vi "TCP Engine Send Loop.vi"(8 "error in (no error)":errorcluster, 11 "Send Loop Notifier":refnum<notifier>) -> (0 "error out":errorcluster)   [LabVIEW 2024, in "TCP Engine.lvlib"]
doc: "This VI will semd all engine response to HOST\n\n\n\nAll Rights Reserved © 2017 SyncSols"
uses:
  TCP Engine.lvlib
  Controls/TCP Engine Send Loop State Machine Data Cluster.ctl
  Controls/TCP Engine Send Loop Data.ctl
  Controls/TCP Engine Send Loop State Machine Cases.ctl
  Main Engine/Controls/Main Engine Q Option.ctl
  Controls/TCP Engine Q Driver Options.ctl
  Controls/TCP Engine State Machine Cases.ctl
panel:
  in  "Data Cluster":T1
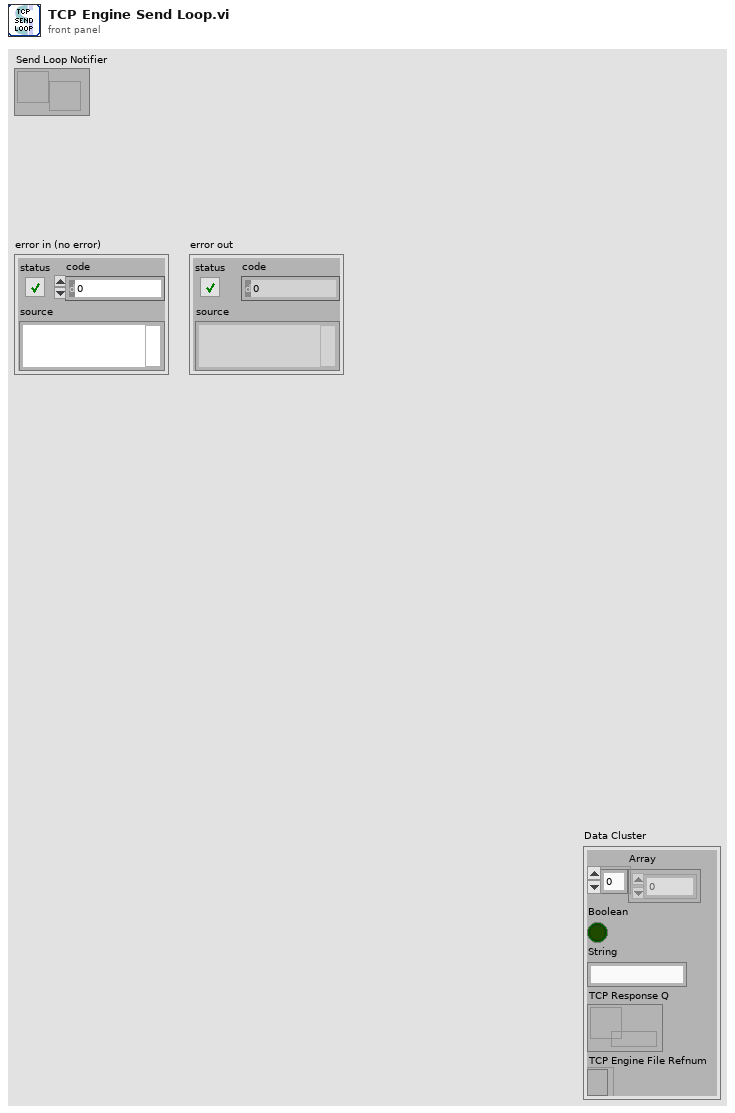
[diagram p1: front panel]
types:
  T1 = typedef "TCP Engine.lvlib/TCP Engine Send Loop State Machine Data Cluster.ctl" = cluster{"Array":dbl[], "Boolean":bool, "String":string, "TCP Response Q":refnum<queue>, "TCP Engine File Refnum":refnum<file>}
  T2 = typedef "TCP Engine.lvlib/TCP Engine Send Loop State Machine Cases.ctl" = enum16{">Poll", ".........State Machine.........", ">Init", ">Error", ">Exit", ".........TCP Send Loop..........", ">Send TCP Response"}
  T3 = typedef "Main Engine Q Option.ctl" = enum16{"Init", "Get"}
  T4 = typedef "TCP Engine.lvlib/TCP Engine Q Driver Options.ctl" = enum16{"Initialize", "EnQ", "DeQ", "EnQ at Opp", "Get Q Status", "Flush Q", "Release Q"}
  T5 = enum16{"big-endian, network order", "native, host order", "little-endian"}
  T6 = typedef "TCP Engine.lvlib/TCP Engine Send Loop Data.ctl" = cluster{"Start Send Loop":bool, "Stop Send Loop":bool, "Connection ID":refnum<k5>[], "Log File Path":path}
  T7 = typedef "TCP Engine.lvlib/TCP Engine State Machine Cases.ctl" = enum16{">Poll", ".........State Machine.........", ">Init", ">Init Configuration", ">Decode Configuration", ">Error", ">Exit", "..........TCP Engine..........", ">Wait for Listener", ">Get Msg from HOST", ">Decode the Command", ">Create Listerner ID"}
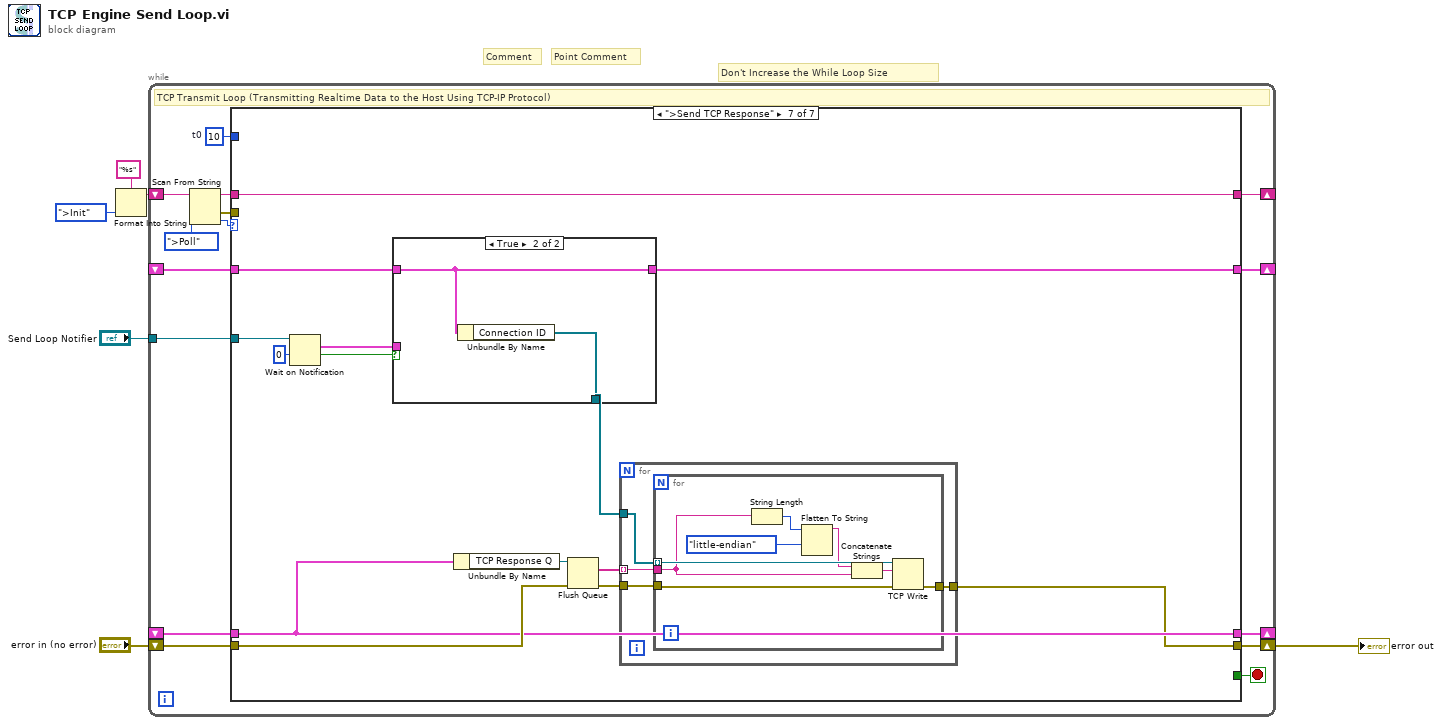
[diagram p0: block diagram]
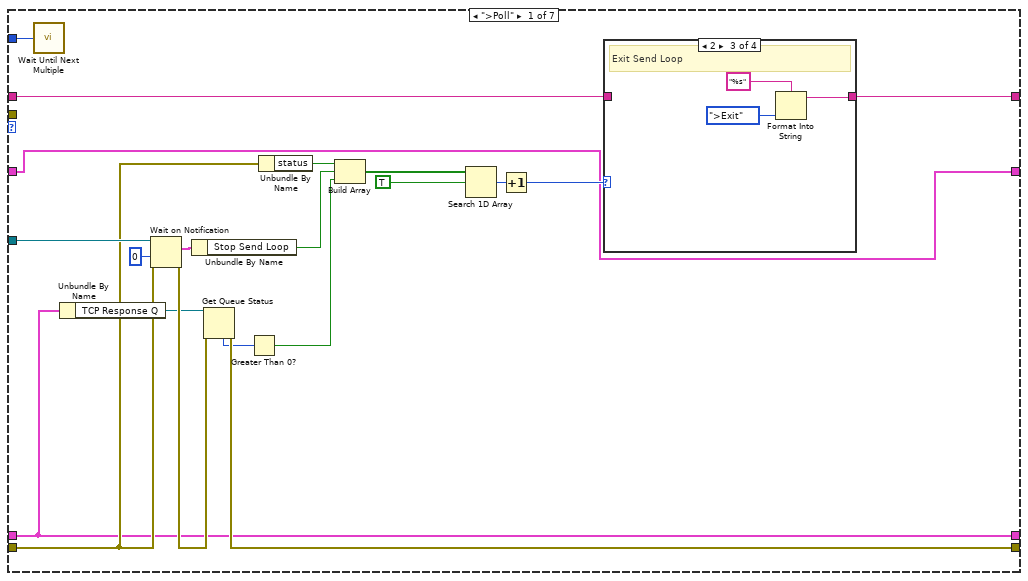
[diagram p2: hidden frame]
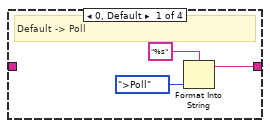
[diagram p3: hidden frame]
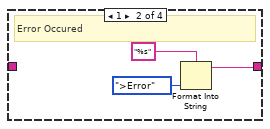
[diagram p4: hidden frame]
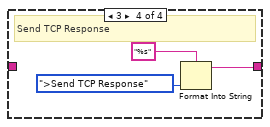
[diagram p5: hidden frame]
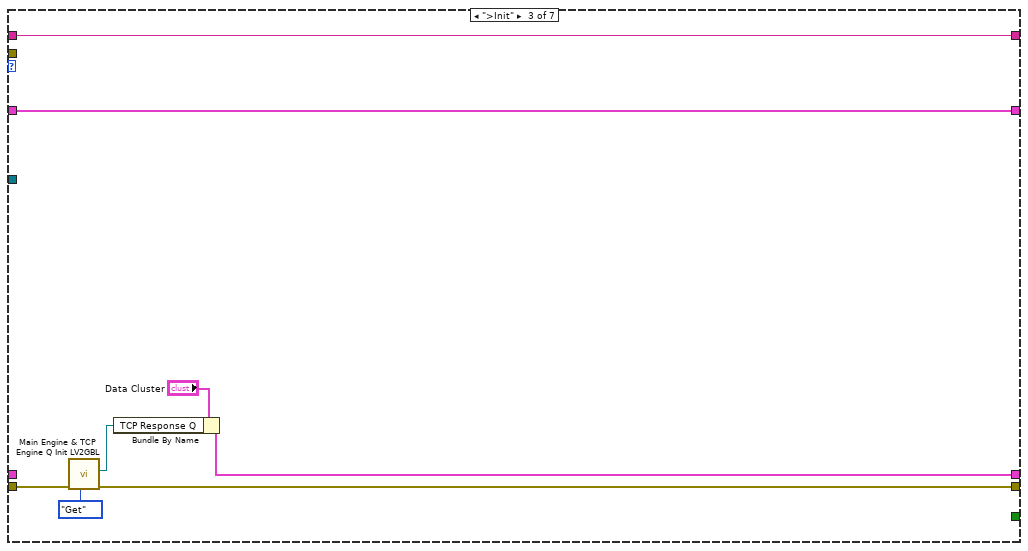
[diagram p7: hidden frame]
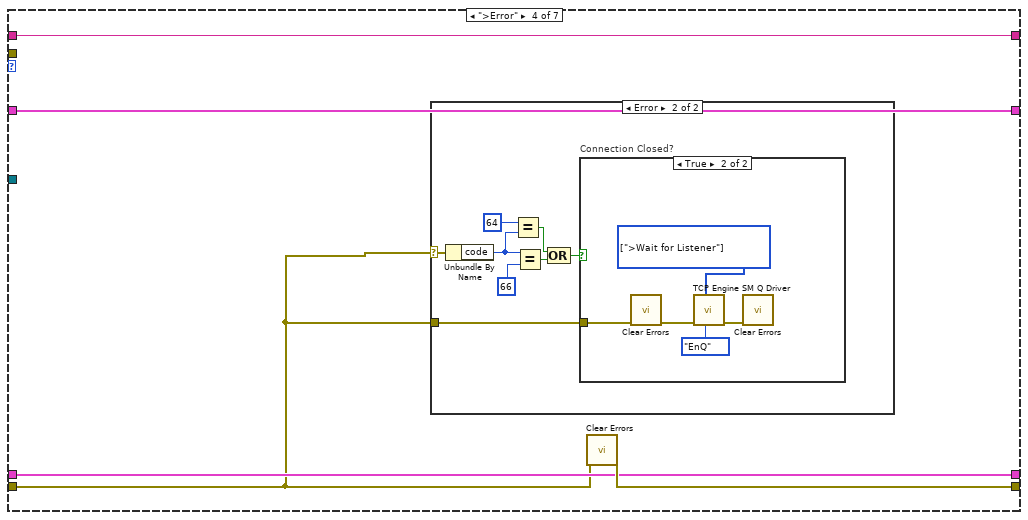
[diagram p8: hidden frame]
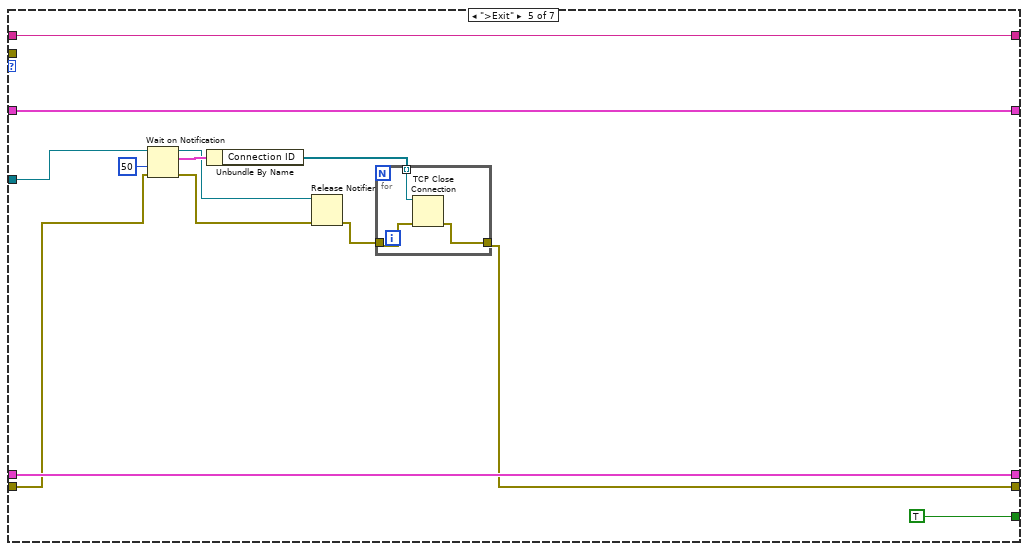
[diagram p11: hidden frame]
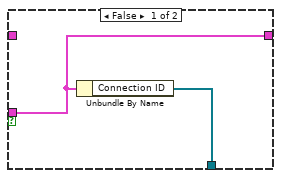
[diagram p13: hidden frame]
diagram:
  # "Don't Increase the While Loop Size"
  # "Point Comment"
  # "Comment"
  n1 = Format Into String(format string="%s", TCP_Engine_Send_Loop_State_Machine_Cases.">Init" ("SM Cases Options")) -> (resulting string=w5:string)  [unwired: 2 in, 1 out]
  n2 = while {
    shift-right: [w16] -> _
    shift-left: w5 -> [w21]
    shift-right: [w14] -> w2
    shift-left: "error in (no error)" -> [w15]
    shift-right: [w12] -> _
    shift-left: _ -> [w11]
    tunnel: "Send Loop Notifier" -> [w9]
    shift-right: [w8] -> _
    shift-left: _ -> [w7]
    stop <- w13 stop-if-true
    w10 = 10  # t0
    # "TCP Transmit Loop (Transmitting Realtime Data to the Host Using TCP-IP Protocol)"
    n3 = Scan From String(input string=w21, default 1=TCP_Engine_Send_Loop_State_Machine_Cases.">Poll" ("SM Cases Options")) -> (remaining string=w17:string, error out=w19:errorcluster, output 1=w18:T2)  [unwired: 3 in, 1 out]
    n4 = case shown="\">Send TCP Response\"" w18 {
      tunnel: w19 -> [_ _ _ _ _ _ _]
      tunnel: w17 -> [w41 w57 w65 w70 w96 w103 w117]
      tunnel: [w40 w57 w65 w70 w96 w103 w117] -> w16
      tunnel: w15 -> [w31 w56 w60 w67 w87 w102 w116]
      tunnel: [w29 w56 w61 w69 w92 w102 w111] -> w14
      tunnel: [_ _ _ _ TRUE _ _] -> w13
      tunnel: [w26 w55 w63 w68 w94 w101 w115] -> w12
      tunnel: w11 -> [w26 w55 _ w68 w94 w101 w115]
      tunnel: w10 -> [w23 _ _ _ _ _ _]
      tunnel: w9 -> [w34 _ _ _ w89 _ w109]
      tunnel: [w22 w54 w58 w66 w84 w100 w105] -> w8
      tunnel: w7 -> [w22 w54 w58 w66 w84 w100 w104]
      frame ">Poll" {
        n5 = call "Wait Until Next Multiple"("Count(mSec)"=w23) -> ()  [unwired: 1 out]
        n6 = Unbundle By Name(w26) -> ("TCP Response Q"=w25:refnum<queue>)
        n7 = Wait on Notification(notifier=w34, timeout in ms (-1)=0, error in (no error)=w31) -> (notification=w33:T6, error out=w30:errorcluster)  [unwired: 1 in, 2 out]
        n8 = Unbundle By Name(w33) -> ("Stop Send Loop"=w32:bool)
        n9 = Get Queue Status(queue=w25, error in (no error)=w30) -> (error out=w29:errorcluster, # elements in queue=w28:i32)  [unwired: 1 in, 6 out]
        n10 = Greater Than 0?(x=w28) -> (x > 0?=w27:bool)
        n11 = Unbundle By Name(w31) -> ("status"=w39:bool)
        n12 = Build Array(w39, w32, w27) -> (w38:bool[])
        n13 = Search 1D Array(1D array=w38, element=TRUE) -> (index of element=w36:i32)  [unwired: 1 in]
        n14 = Increment(x=w36) -> (x+1=w35:i32)
        n15 = case shown="2" w35 {
          tunnel: w41 -> [_ _ _ _]
          tunnel: [w42 w45 w48 w51] -> w40
          frame 0, Default {
            # "Default -> Poll"
            n16 = Format Into String(format string="%s", TCP_Engine_Send_Loop_State_Machine_Cases.">Poll" ("SM Cases Options")) -> (resulting string=w42:string)  [unwired: 2 in, 1 out]
          }
          frame 1 {
            # "Error Occured"
            n17 = Format Into String(format string="%s", TCP_Engine_Send_Loop_State_Machine_Cases.">Error" ("SM Cases Options")) -> (resulting string=w45:string)  [unwired: 2 in, 1 out]
          }
          frame 2 {
            # "Exit Send Loop"
            n18 = Format Into String(format string="%s", TCP_Engine_Send_Loop_State_Machine_Cases.">Exit" ("SM Cases Options")) -> (resulting string=w48:string)  [unwired: 2 in, 1 out]
          }
          frame 3 {
            # "Send TCP Response"
            n19 = Format Into String(format string="%s", TCP_Engine_Send_Loop_State_Machine_Cases.">Send TCP Response" ("SM Cases Options")) -> (resulting string=w51:string)  [unwired: 2 in, 1 out]
          }
        }
      }
      frame ".........State Machine........." {
      }
      frame ">Init" {
        n20 = call "Main Engine & TCP Engine Q Init LV2GBL.vi"("Q Option"=Main_Engine_Q_Option."Get", "error in"=w60) -> ("error out"=w61:errorcluster, "TCP Enigine Tx-Q"=w62:refnum<queue>)  [unwired: 7 in, 1 out]
        n21 = Bundle By Name(cluster="Data Cluster", "TCP Response Q"=w62) -> (w63:T1)
      }
      frame ">Error" {
        n22 = case shown="Error" w67 {
          selector: w67 -> [_ w78]
          tunnel: w67 -> [_ w76]
          frame No Error {
          }
          frame Error {
            n23 = Unbundle By Name(w78) -> ("code"=w74:i32)
            n24 = Equal?(x=64, y=w74) -> (x = y?=w75:bool)
            n25 = Equal?(x=w74, y=66) -> (x = y?=w72:bool)
            n26 = Compound Arithmetic op=OR(w75, w72) -> (w71:bool)
            n27 = case "Connection Closed?" shown="True" w71 {
              tunnel: w76 -> [_ w80]
              frame False {
              }
              frame True {
                w82 = T7[] [enum.">Wait for Listener"] items=[">Poll", ".........State Machine.........", ">Init", ">Init Configuration", ">Decode Configuration", ">Error", ">Exit", "..........TCP Engine..........", ">Wait for Listener", ">Get Msg from HOST", ">Decode the Command", ">Create Listerner ID"] ("States")
                n28 = call <vilib>:"Clear Errors.vi"("error in (no error)"=w80) -> ("error out"=w81:errorcluster)  [unwired: 5 in, 1 out]
                n29 = call "TCP Engine SM Q Driver.vi"("Q Driver Options"=TCP_Engine_Q_Driver_Options."EnQ", "States"=w82, "error in"=w81) -> ("error out"=w79:errorcluster)  [unwired: 4 in, 4 out]
                n30 = call <vilib>:"Clear Errors.vi"("error in (no error)"=w79) -> ()  [unwired: 5 in, 2 out]
              }
            }
          }
        }
        n31 = call <vilib>:"Clear Errors.vi"("error in (no error)"=w67) -> ("error out"=w69:errorcluster)  [unwired: 5 in, 1 out]
      }
      frame ">Exit" {
        n32 = Wait on Notification(notifier=w89, timeout in ms (-1)=50, error in (no error)=w87) -> (notifier out=w88:refnum<notifier>, notification=w90:T6, error out=w86:errorcluster)  [unwired: 1 in, 1 out]
        n33 = Unbundle By Name(w90) -> ("Connection ID"=w85:refnum<k5>[])
        n34 = Release Notifier(notifier=w88, error in (no error)=w86) -> (error out=w93:errorcluster)  [unwired: 1 in, 2 out]
        n35 = for {
          tunnel: w93 -> [w99]
          tunnel: [w98] -> w92
          tunnel: w85 -> [w97] mode=indexing
          n36 = TCP Close Connection(connection ID=w97, error in (no error)=w99) -> (error out=w98:errorcluster)  [unwired: 1 in, 1 out]
        }
      }
      frame ".........TCP Send Loop.........." {
      }
      frame ">Send TCP Response" {
        n37 = Wait on Notification(notifier=w109, timeout in ms (-1)=0) -> (notification=w107:T6, timed out?=w108:bool)  [unwired: 2 in, 2 out]
        n38 = case shown="True" w108 {
          tunnel: w104 -> [_ w121]
          tunnel: w107 -> [w118 _]
          tunnel: [w119 w120] -> w106
          tunnel: [w118 w121] -> w105
          frame False {
            n39 = Unbundle By Name(w118) -> ("Connection ID"=w119:refnum<k5>[])
          }
          frame True {
            n40 = Unbundle By Name(w121) -> ("Connection ID"=w120:refnum<k5>[])
          }
        }
        n41 = Unbundle By Name(w115) -> ("TCP Response Q"=w114:refnum<queue>)
        n42 = Flush Queue(queue=w114, error in (no error)=w116) -> (remaining elements=w112:string[], error out=w113:errorcluster)  [unwired: 1 out]
        n43 = for {
          tunnel: w106 -> [w124]
          tunnel: w113 -> [w125]
          tunnel: w112 -> [w122] mode=indexing
          tunnel: [w123] -> w111
          n44 = for {
            tunnel: w124 -> [w132] mode=indexing
            tunnel: w122 -> [w129]
            tunnel: w125 -> [w126]
            tunnel: [w131] -> w123
            n45 = String Length(string=w129) -> (length=w133:i32)
            n46 = Flatten To String(anything=w133, byte order (0:big-endian, network order)=T5."little-endian") -> (data string=w130:string)  [unwired: 2 in, 2 out]
            n47 = Concatenate Strings(w130, w129) -> (w128:string)
            n48 = TCP Write(connection ID=w132, data in=w128, error in (no error)=w126) -> (error out=w131:errorcluster)  [unwired: 1 in, 2 out]
          }
        }
      }
    }
  }
  "error out" <- w2
